vi "Build Filter Configuration.vi"(7 "Virtual Memory Unit in":refnum<class "Virtual Memory Unit.lvclass">, 8 "error in (no error)":errorcluster, 10 "Simple Mode (Blacklist)":bool, 11 "Filter in":refnum<class "Filter.lvclass">) -> (0 "error out":errorcluster, 5 "Virtual Memory Unit out":refnum<class "Virtual Memory Unit.lvclass">)   [LabVIEW 2020, in "BCI-1553 API.lvlib" / "Filter.lvclass"]
doc: "<DO NOT CALL>\n\nThis method is leveraged by the Bus Monitor to produce the raw configuration values for setting up a filter in hardware."
uses:
  Filter.lvclass
  Dependencies/Virtual Memory Unit/Virtual Memory Unit.lvclass
  Frames & Messages/TypeDefs/Command Type.ctl
  Filter.lvclass/Filter.ctl
  BCI-1553 API.lvlib
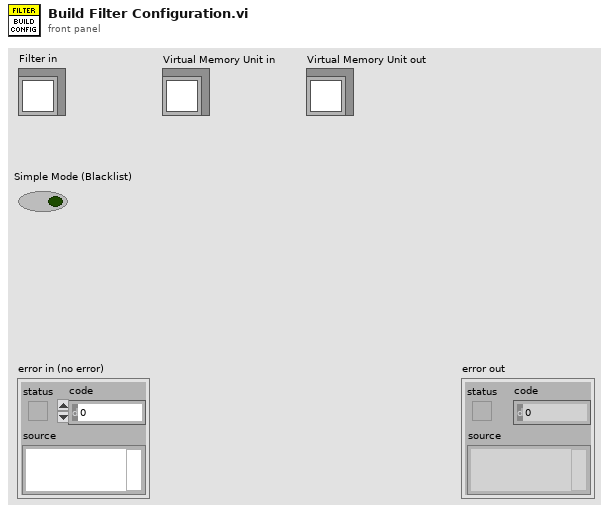
[diagram p1: front panel]
types:
  T1 = typedef "BCI-1553 API.lvlib/Command Type.ctl" = enum16{"Transmit", "Receive"}
  T2 = typedef "BCI-1553 API.lvlib/Command SubAddress.ctl" = enum16{"Mode Code", "1", "2", "3", "4", "5", "6", "7", "8", "9", "10", "11", "12", "13", "14", "15", "16", "17", "18", "19", "20", "21", "22", "23", "24", "25", "26", "27", "28", "29", "30"}
  T3 = typedef "BCI-1553 API.lvlib/Command Terminal Address.ctl" = enum16{"0", "1", "2", "3", "4", "5", "6", "7", "8", "9", "10", "11", "12", "13", "14", "15", "16", "17", "18", "19", "20", "21", "22", "23", "24", "25", "26", "27", "28", "29", "30", "Broadcast"}
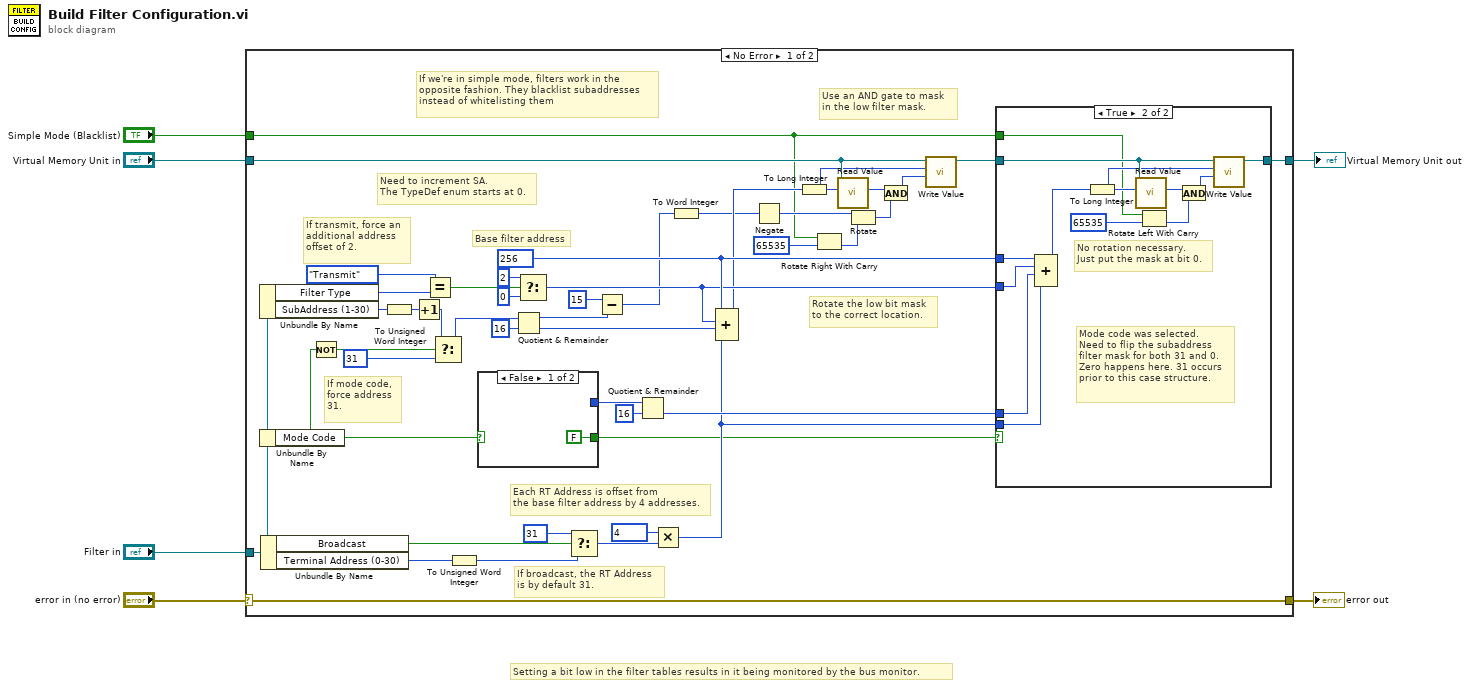
[diagram p0: block diagram]
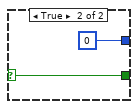
[diagram p3: hidden frame]
diagram:
  # "Setting a bit low in the filter tables results in it being monitored by the bus monitor."
  n1 = case shown="No Error" "error in (no error)" {
    selector: "error in (no error)" -> [w51 w70]
    tunnel: [w51 w70] -> w5
    tunnel: "Filter in" -> [w45 _]
    tunnel: "Virtual Memory Unit in" -> [w23 w69]
    tunnel: [w25 w69] -> w2
    tunnel: "Simple Mode (Blacklist)" -> [w10 _]
    frame No Error {
      w30 = u16 256
      # "Need to increment SA.\nThe TypeDef enum starts at 0."
      # "If we're in simple mode, filters work in the\nopposite fashion. They blacklist subaddresses\ninstead of whitelisting them"
      # "Use an AND gate to mask\nin the low filter mask."
      # "Rotate the low bit mask\nto the correct location."
      # "If transmit, force an\nadditional address\noffset of 2."
      # "If mode code,\nforce address\n31."
      # "Each RT Address is offset from\nthe base filter address by 4 addresses."
      # "If broadcast, the RT Address\nis by default 31."
      # "Base filter address"
      n2 = Unbundle By Name(w45) -> ("Filter Type"=w38:T1, "SubAddress (1-30)"=w42:T2)
      n3 = Unbundle By Name(w45) -> ("Mode Code"=w40:bool)
      n4 = Unbundle By Name(w45) -> ("Broadcast"=w49:bool, "Terminal Address (0-30)"=w50:T3)
      n5 = Not(x=w40) -> (.not. x?=w44:bool)
      n6 = To Unsigned Word Integer(number=w42) -> (unsigned 16bit integer=w9:u16)
      n7 = Increment(x=w9) -> (x+1=w7:u16)
      n8 = Equal?(x=Command_Type."Transmit", y=w38) -> (x = y?=w36:bool)
      n9 = Select(t=w7, s=w44, f=u16 31) -> (s? t:f=w41:u16)
      n10 = To Unsigned Word Integer(number=w50) -> (unsigned 16bit integer=w8:u16)
      n11 = case shown="False" w40 {
        selector: w40 -> [_ w68]
        tunnel: [FALSE w68] -> w26
        tunnel: [_ u16 0] -> w31
        frame False {
        }
        frame True {
        }
      }
      n12 = Quotient & Remainder(x=w41, y=u16 16) -> (x-y*floor(x/y)=w16:u16, floor(x/y)=w33:u16)
      n13 = Select(t=u16 2 ("y"), s=w36, f=u16 0 ("y")) -> (s? t:f=w29:u16)
      n14 = Select(t=u16 31, s=w49, f=w8) -> (s? t:f=w47:u16)
      n15 = Subtract(x=u16 15 ("y"), y=w16) -> (x-y=w14:u16)
      n16 = Quotient & Remainder(x=w31, y=u16 16) -> (floor(x/y)=w28:u16)  [unwired: 1 out]
      n17 = Multiply(x=u16 4, y=w47) -> (x*y=w27:u16)
      n18 = To Word Integer(number=w14) -> (16bit integer=w12:i16)
      n19 = Compound Arithmetic op=ADD(w30, w29, w33, w27) -> (w24:u16)
      n20 = Negate(x=w12) -> (-x=w11:i16)
      n21 = To Long Integer(number=w24) -> (32bit integer=w21:i32)
      n22 = Rotate Right With Carry(2:u16 65535, 3:w10) -> (0:w17:u16)  [unwired: 1 out]
      n23 = call "Read Value.vi"("Index"=w21, "Virtual Memory Unit in"=w23) -> ("Value"=w20:u16)  [unwired: 8 in, 1 out]
      n24 = Rotate(1:w17, 2:w11) -> (0:w13:u16)
      n25 = And(x=w20, y=w13) -> (x .and. y?=w19:u16)
      n26 = call "Write Value.vi"("Value"=w19, "Index"=w21, "Virtual Memory Unit in"=w23) -> ("Virtual Memory Unit out"=w22:refnum<class "Virtual Memory Unit.lvclass">)  [unwired: 7 in, 1 out]
      n27 = case shown="True" w26 {
        tunnel: w30 -> [_ w65]
        tunnel: w29 -> [_ w64]
        tunnel: w28 -> [_ w63]
        tunnel: w27 -> [_ w62]
        tunnel: w22 -> [w52 w60]
        tunnel: [w52 w59] -> w25
        tunnel: w10 -> [_ w53]
        frame False {
          # "Not mode code. Don't flip another bit low."
        }
        frame True {
          # "No rotation necessary.\nJust put the mask at bit 0."
          # "Mode code was selected.\nNeed to flip the subaddress\nfilter mask for both 31 and 0.\nZero happens here. 31 occurs\nprior to this case structure."
          n28 = Compound Arithmetic op=ADD(w65, w64, w63, w62) -> (w61:u16)
          n29 = To Long Integer(number=w61) -> (32bit integer=w58:i32)
          n30 = call "Read Value.vi"("Index"=w58, "Virtual Memory Unit in"=w60) -> ("Value"=w56:u16)  [unwired: 8 in, 1 out]
          n31 = Rotate Left With Carry(2:u16 65535, 3:w53) -> (0:w55:u16)  [unwired: 1 out]
          n32 = And(x=w56, y=w55) -> (x .and. y?=w54:u16)
          n33 = call "Write Value.vi"("Value"=w54, "Index"=w58, "Virtual Memory Unit in"=w60) -> ("Virtual Memory Unit out"=w59:refnum<class "Virtual Memory Unit.lvclass">)  [unwired: 7 in, 1 out]
        }
      }
    }
    frame Error {
    }
  }
  "error out" <- w5
  "Virtual Memory Unit out" <- w2
